vi "errorhandler.vi"(0 "HGF_SVMonitor in":refnum<class "HGF_SVMonitor.lvclass">, 5 "Error Array":errorcluster[](array[cluster])) -> (14 "HGF_SVMonitor out":refnum<class "HGF_SVMonitor.lvclass">, 19 "error out":errorcluster)   [LabVIEW 2012, in "HGF_SV.lvlib" / "HGF_SVMonitor.lvclass"]
doc: "Error handling for the HGF_SVMonitor class."
uses:
  HGF_SVMonitor.lvclass
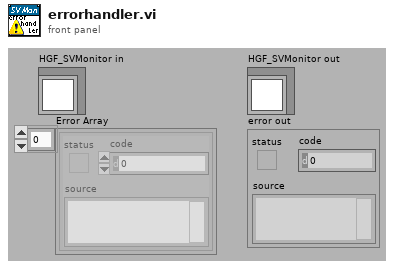
[diagram p1: front panel]
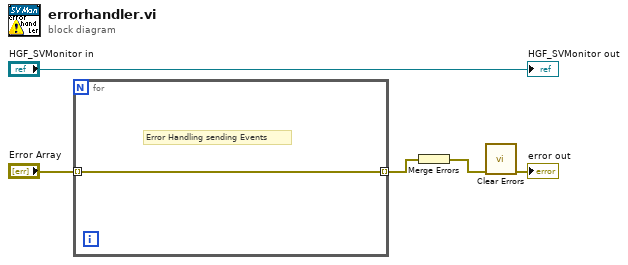
[diagram p0: block diagram]
diagram:
  n1 = for {
    tunnel: "Error Array" -> [w6] mode=indexing
    tunnel: [w6] -> w3 mode=indexing
    # "Error Handling sending Events"
  }
  n2 = Merge Errors(w3) -> (w2:errorcluster)
  n3 = call <vilib>:"Clear Errors.vi"("error in (no error)"=w2) -> ("error out"=→"error out":errorcluster)  [unwired: 6 out]
  "HGF_SVMonitor out" <- "HGF_SVMonitor in"
